vi "OE1201_Configure Channel Out.vi"(7 "OE1201_Configure Channel Out":T1={"CH 1"=3, "CH 2"=3, "CH2 Offset(%)"=0.0, "CH1 Offset(%)"=0.0, "CH2 Expand"=1, "CH1 Expand"=1} {"CH1 Expand" min=1 max=256; "CH2 Expand" min=1 max=256; "CH1 Offset(%)" min=-100.0 max=100.0 format="%#.2g"; "CH2 Offset(%)" min=-100.0 max=100.0 format="%#.2g"; "CH 2" items=["R"=3, "X"=1, "Y"=2, "θ"=4]; "CH 1" items=["R"=3, "X"=1, "Y"=2, "θ"=4]}, 8 "Error in (no error)":errorcluster caption="error out（no error）", 9 "Remote Mode":u16(ring) items=["USB", "RS232"], 11 "VISA resource name":refnum<visa-resource-name>) -> (0 "Error out":errorcluster caption="error out", 1 "Output String":string, 3 "VISA resource  out":refnum<visa-resource-name>)   [LabVIEW 2011]
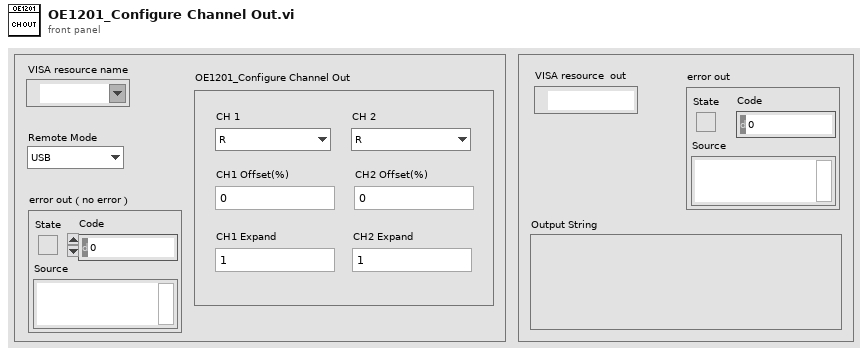
[diagram p1: front panel]
types:
  T1 = cluster{"CH 1":i8, "CH 2":i8, "CH2 Offset(%)":dbl, "CH1 Offset(%)":dbl, "CH2 Expand":u16, "CH1 Expand":u16}
  T2 = enum16{"ISRC", "IGND", "ICPL", "ILIN", "PHAS", "FMOD", "RSLP", "FREQ", "SWPT", "SLLM", "SULM", "SSLL", "SSLG", "STLM", "SWRM", "IRNG", "SENS", "RMOD", "OFLT", "OFSL", "SYNC", "DMOD", "HARM", "DARB", "SWVT", "SLVL", "SVLL", "SVUL", "SVSL", "SVSG", "SVTM", "SVRM", "RALL", "SNAP", "OUTP", "OAUX", "COUT", "CAUX", "COFP", "CEXP", "FPOP", "OEXP", "*IDN", "*RST", "OVLD", "INOV", "GNOV", "*PLL", "SSET", "RSET", "AGAN", "APHS", "ARSV", "ASCL", "EQCD", "EQCS", "SPED", "SRAT", "SLEN", "SSLE", "STRG", "SPRM", "STRD", "PAUS", "REST", "SPTS", "TRCA", "TEMP", "RSTU", "IHNZ", "DEQU", "SADD", "ARNG", "CSPE", "ISRCD", "IGNDD", "ICPLD", "ILIND", "PHASD", "FMODD", "RSLPD", "FREQD", "SWPTD", "SLLMD", "SULMD", "SSLLD", "SSLGD", "STLMD", "SWRMD", "SENSD", "RMODD", "OFLTD", "OFSLD", "SYNCD", "HARMD", "EQCDD", "EQCSD", "SNAPD", "OUTPD", "SWVTD", "SLVLD", "SVLLD", "SVULD", "SVSLD", "SVSGD", "SVTMD", "SVRMD", "SVDCD", "ARSVD", "AGAND", "APHSD", "ASCLD", "FPOPD", "CAUXD", "OEXPD", "SPEDD", "SRATD", "SLEND", "SSLED", "STRGD", "SPRMD", "STRDD", "PAUSD", "RESTD", "SPTSD", "TRCAD", "*IDND", "*RSTD", "INOVD", "GNOVD", "*PLLD", "SSETD", "RSETD"}
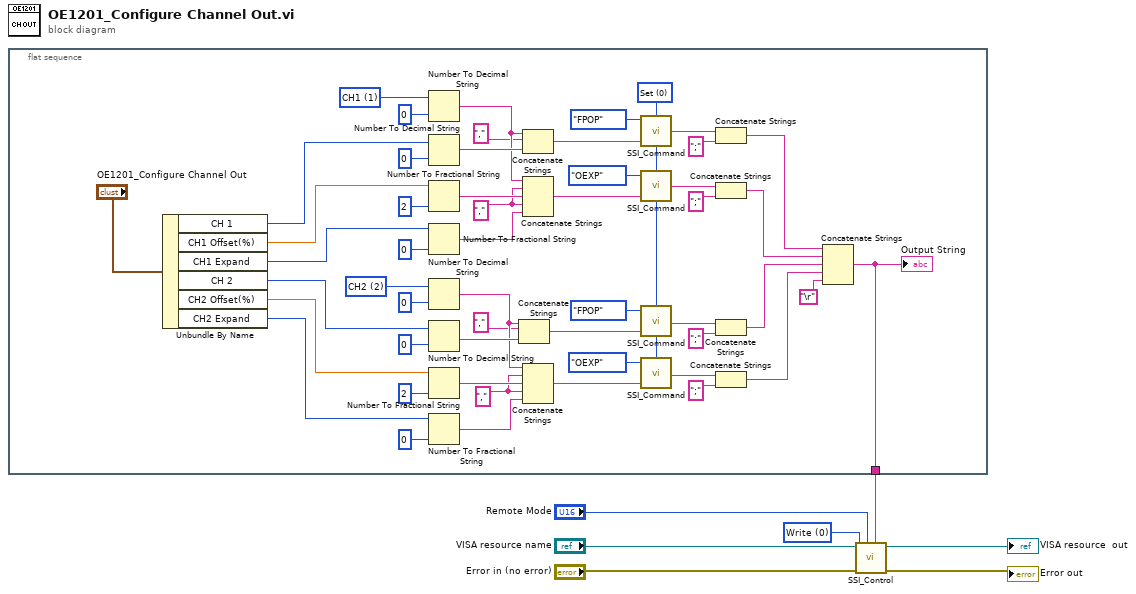
[diagram p0: block diagram]
diagram:
  w6 = u16 0 items=["Write", "Read"] ("Control")
  n1 = flat-sequence {
    tunnel: [w59] -> w1
    frame #0 {
      w12 = ","
      w23 = ","
      w29 = u16 2 items=["CH1"=1, "CH2"=2]
      w28 = u16 1 items=["CH1"=1, "CH2"=2]
      w41 = u16 0 items=["Set", "Query"] ("Opera")
      n2 = Unbundle By Name("OE1201_Configure Channel Out") -> ("CH 1"=w38:i8, "CH1 Offset(%)"=w11:dbl, "CH1 Expand"=w10:u16, "CH 2"=w37:i8, "CH2 Offset(%)"=w9:dbl, "CH2 Expand"=w8:u16)
      n3 = Number To Decimal String(number=w28, width (-)=i16 0 ("精度(6)")) -> (decimal integer string=w25:string)
      n4 = Number To Decimal String(number=w38, width (-)=i16 0 ("精度(6)")) -> (decimal integer string=w27:string)
      n5 = Number To Fractional String(number=w11, precision (6)=i16 2 ("精度(6)")) -> (F-format string=w24:string)  [unwired: 2 in]
      n6 = Number To Fractional String(number=w10, precision (6)=i16 0 ("精度(6)")) -> (F-format string=w22:string)  [unwired: 2 in]
      n7 = Number To Decimal String(number=w29, width (-)=i16 0 ("精度(6)")) -> (decimal integer string=w20:string)
      n8 = Number To Decimal String(number=w37, width (-)=i16 0 ("精度(6)")) -> (decimal integer string=w21:string)
      n9 = Number To Fractional String(number=w9, precision (6)=i16 2 ("精度(6)")) -> (F-format string=w19:string)  [unwired: 2 in]
      n10 = Number To Fractional String(number=w8, precision (6)=i16 0 ("精度(6)")) -> (F-format string=w18:string)  [unwired: 2 in]
      n11 = Concatenate Strings(w20, ",", w21) -> (w16:string)
      n12 = Concatenate Strings(w25, ",", w27) -> (w26:string)
      n13 = Concatenate Strings(w25, w23, w24, w23, w22) -> (w15:string)
      n14 = Concatenate Strings(w20, w12, w19, w12, w18) -> (w17:string)
      n15 = call "SSI_Command.vi"("Opera"=w41, "Paramter"=w26, "Command Type"=T2."FPOP") -> ("Output string"=w48:string)  [unwired: 1 in]
      n16 = call "SSI_Command.vi"("Opera"=w41, "Paramter"=w15, "Command Type"=T2."OEXP") -> ("Output string"=w52:string)  [unwired: 1 in]
      n17 = call "SSI_Command.vi"("Opera"=w41, "Paramter"=w16, "Command Type"=T2."FPOP") -> ("Output string"=w50:string)  [unwired: 1 in]
      n18 = call "SSI_Command.vi"("Opera"=w41, "Paramter"=w17, "Command Type"=T2."OEXP") -> ("Output string"=w42:string)  [unwired: 1 in]
      n19 = Concatenate Strings(w48, ";" ("替换字符串(\"\")")) -> (w36:string)
      n20 = Concatenate Strings(w52, ";" ("替换字符串(\"\")")) -> (w35:string)
      n21 = Concatenate Strings(w50, ";" ("替换字符串(\"\")")) -> (w34:string)
      n22 = Concatenate Strings(w42, ";" ("替换字符串(\"\")")) -> (w33:string)
      n23 = Concatenate Strings(w36, w35, w34, w33, "\r") -> (w59:string)
      "Output String" <- w59
    }
  }
  n24 = call "SSI_Control.vi"("Write Buffer"=w1, "Remote Mode"="Remote Mode", "Error in (no error)"="Error in (no error)", "Control"=w6, "VISA resource name"="VISA resource name") -> ("Error out"=→"Error out":errorcluster, "VISA resource  out"=→"VISA resource  out":refnum<visa-resource-name>)  [unwired: 3 in, 2 out]
